vi "tfyghj.vi"() -> ()   [LabVIEW 2021]
uses:
  <vilib>/Platform/TimedLoop/XDataNode/timing_clust.ctl
  <vilib>/Platform/TimedLoop/XDataNode/nitl_modes.ctl
  <vilib>/Platform/TimedLoop/XDataNode/wakeup.ctl
  <vilib>/rvi/Emulation/niFpgaGetClockAttributes.vi
  <vilib>/rvi/Emulation/niFpgaSctlEmulationGetInTimedLoop.vi
  <vilib>/rvi/Emulation/niFpgaEmulationReportErrorSimple.vi
  <vilib>/rvi/Emulation/niFpgaCriticalErrorInLSC.vi
  <vilib>/platform/TimedLoop/XDataNode/XDataNode.xnode
  <vilib>/Platform/TimedLoop/XDataNode/XDNodeRunTimeDep.lvlib
panel:
  out "lut value at index":i16
  in  "Math":bool
  in  "PUT DIFFERENCE":i32
  out "Saw tooth \nactual freq":fxp<+,32,16>
  out "needed pre conversion":fxp<+,32,16>
  in  "Frequency":i32
  out "ticks needed post conversion":fxp<+/-,64,34>
  in  "SET DESIRED TICK":u32
  in  "Sin":bool
  out "sine out 3":i16
  out "sine out 2":i16
  out "sine out":i16
  out "C":bool
  out "B":bool
  out "Index":i32
  out "Difference Between":u32
  out "Current Time":u32
  out "Previous Time":u32
  out "A":bool
  out "Tick Count(Ticks)":u32
  in  "main":bool
  # "HOW TO USE:\n1) set desired SIN frequency\n2) the outputted ticks needed will be provided \nto find a frequency for the sawtooth ath is minimum 15x greater!\n!!!\nIF YOU PUT A DESIRED TICK SMALLER THAN THE NEEDED IT WILL\nPROVIDE A HIGHER FREQUENCY , A LARGER WILL BE SMALLER\n!!!"
  # "This is to calculate the actual frequency, put inside the difference\nto see what our lookup tabe output is actualy being worked at"
  # "IGNORE FOR NOW!!! HAVENT IMPLEMENTED\nchecks comparison of carrier and sin"
  # "This just reads out \nvalues from sin wave"
  # "Checks index and LUT values"
  # "WHere difference is derived"
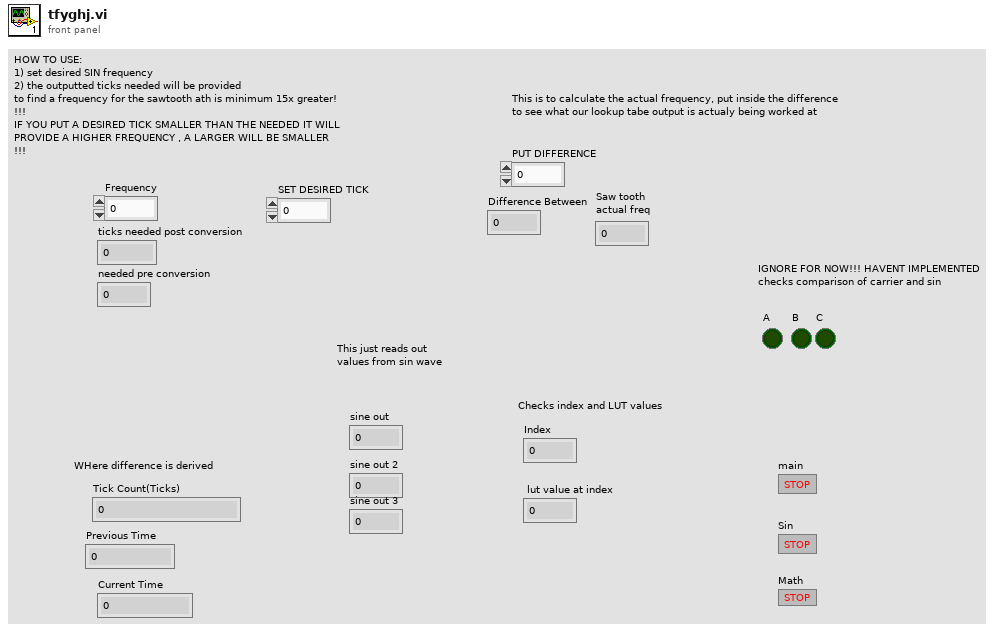
[diagram p1: front panel]
types:
  T1 = typedef "XDNodeRunTimeDep.lvlib/timing_clust.ctl" = cluster{"Expected End [f-1]":u64, "Actual End [f-1]":u64, "Finished Late? [f-1]":bool, "Expected End [i-1]":u64, "Actual End [i-1]":u64, "Finished Late? [i-1]":bool, "Expected Start [i]":u64, "Actual Start [i]":u64, "Expected Start [f]":u64, "Actual Start [f]":u64, "Source Name":string, "Structure Name":string, "Period":i64, "Deadline":i64, "Offset":i64, "Start":i64, "Priority":i32, "Timeout":i32, "Mode":T2, "Wakeup Reason":T3, "Error":errorcluster, "Source Type":string, "Secondary Source Type":string, "Global End Time":u64, "Global Start Time":u64, "Frame Duration":u64, "Iteration Duration":u64, "Assigned CPU":i32, "I/O Scan Engine Mode":u32}
  T2 = typedef "XDNodeRunTimeDep.lvlib/nitl_modes.ctl" = enum32{"No Change", "Process missed periods, maintain original phase", "Discard missed periods, maintain original phase", "Process missed periods, ignore original phase", "Discard missed periods, ignore original phase"}
  T3 = typedef "XDNodeRunTimeDep.lvlib/wakeup.ctl" = enum32{"Normal", "Aborted", "Asynchronous wakeup", "Timing source error", "Timed loop error", "Timeout"}
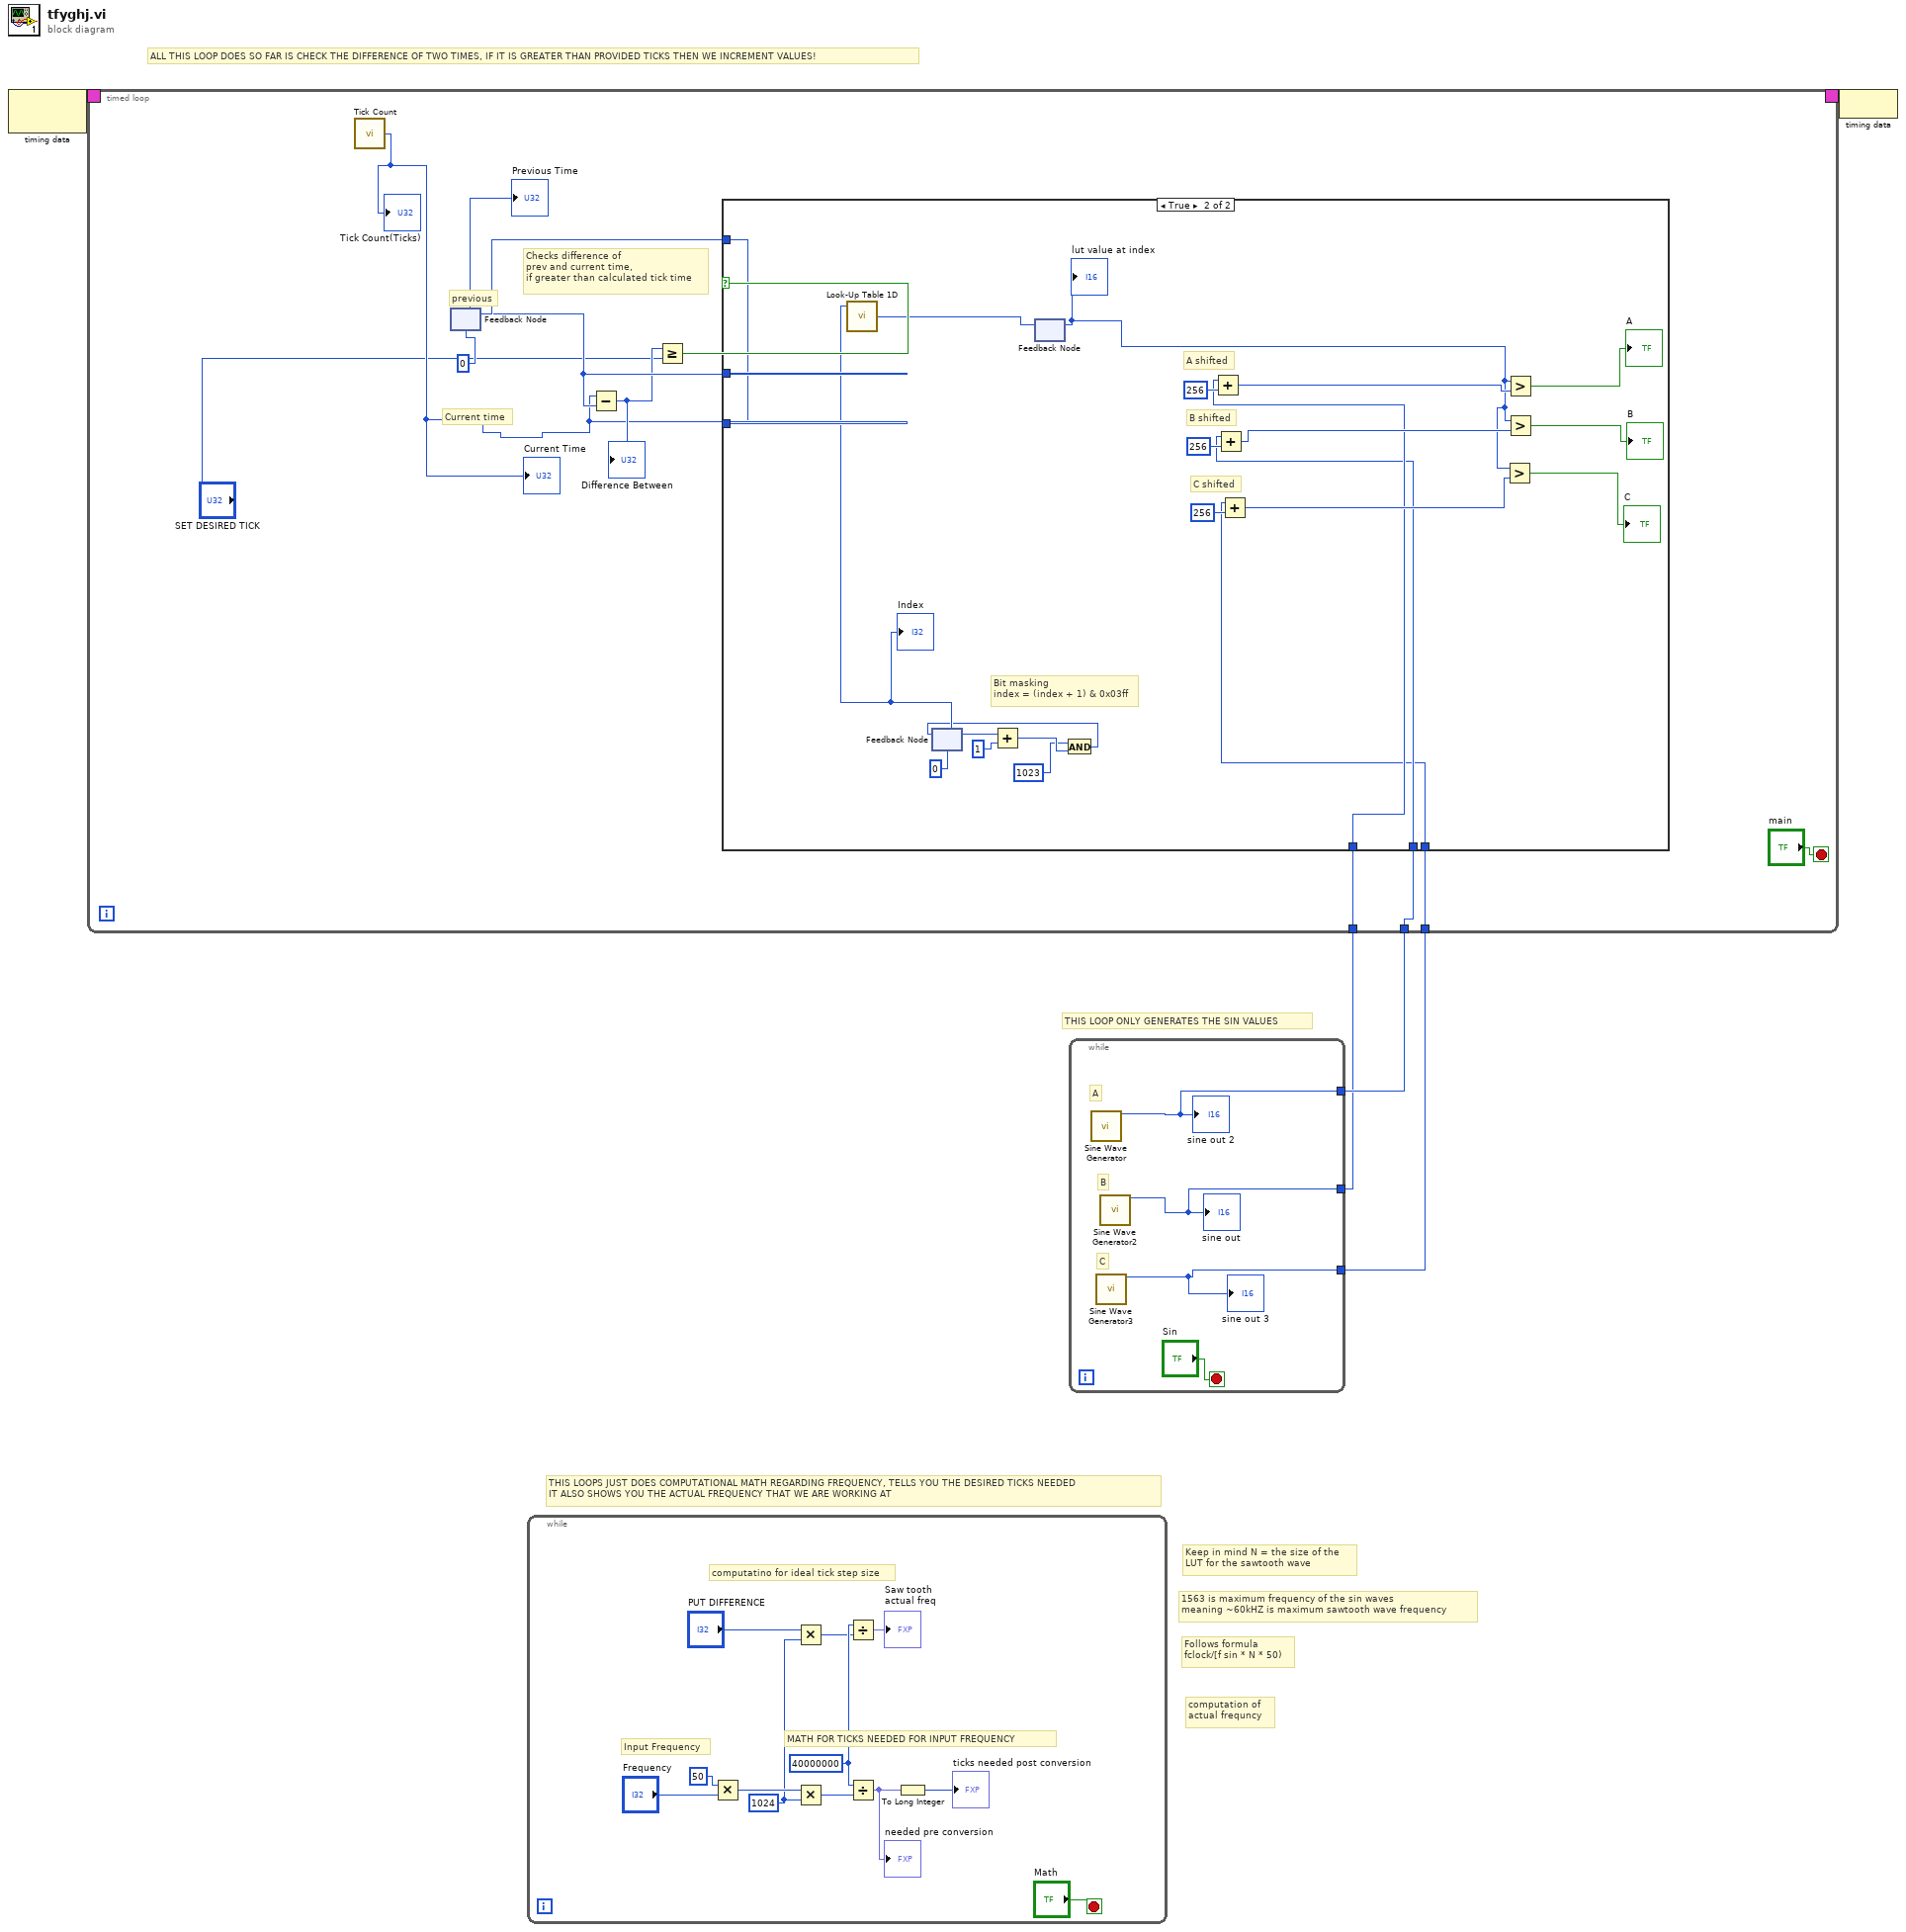
[diagram p0: block diagram]
diagram:
  # "ALL THIS LOOP DOES SO FAR IS CHECK THE DIFFERENCE OF TWO TIMES, IF IT IS GREATER THAN PROVIDED TICKS THEN WE INCREMENT VALUES!"
  # "computation of \nactual frequncy"
  # "1563 is maximum frequency of the sin waves \nmeaning ~60kHZ is maximum sawtooth wave frequency"
  # "Keep in mind N = the size of the \nLUT for the sawtooth wave"
  # "Follows formula \nfclock/[f sin * N * 50)"
  # "THIS LOOPS JUST DOES COMPUTATIONAL MATH REGARDING FREQUENCY, TELLS YOU THE DESIRED TICKS NEEDED\nIT ALSO SHOWS YOU THE ACTUAL FREQUENCY THAT WE ARE WORKING AT"
  # "THIS LOOP ONLY GENERATES THE SIN VALUES"
  n1 = node-c288() -> (w5:T1)  [unwired: 1 in]
  n2 = while {
    stop <- "Math" stop-if-true
    w11 = 1024
    w12 = 40000000
    # "MATH FOR TICKS NEEDED FOR INPUT FREQUENCY"
    # "computatino for ideal tick step size"
    # "Input Frequency"
    n3 = Multiply(x=50, y="Frequency") -> (x*y=w16:i32)
    n4 = Multiply(x="PUT DIFFERENCE", y=w11) -> (x*y=w10:u32)
    n5 = Multiply(x=w16, y=w11) -> (x*y=w15:i32)
    n6 = Divide(x=w12, y=w10) -> (x/y=→"Saw tooth \nactual freq":fxp<+,32,16>)
    n7 = Divide(x=w12, y=w15) -> (x/y=w14:fxp<+,32,16>)
    "needed pre conversion" <- w14
    n8 = To Long Integer(number=w14) -> (32bit integer=→"ticks needed post conversion":i32)
  }
  n9 = while {
    tunnel: [w20] -> w3
    tunnel: [w19] -> w2
    tunnel: [w18] -> w1
    stop <- "Sin" stop-if-true
    # "C"
    # "A"
    # "B"
    n10 = call "Sine Wave Generator"() -> ("sine out"=w20:i16)  [unwired: 15 in]
    "sine out 2" <- w20
    n11 = call "Sine Wave Generator3"() -> ("sine out"=w18:i16)  [unwired: 15 in]
    "sine out 3" <- w18
    n12 = call "Sine Wave Generator2"() -> ("sine out"=w19:i16)  [unwired: 15 in]
    "sine out" <- w19
  }
  n13 = timed-loop {
    timing: w5 -> [_]
    timing-out: [_] -> w4
    tunnel: w3 -> [w23]
    tunnel: w2 -> [w24]
    tunnel: w1 -> [w22]
    stop <- "main" stop-if-true
    # "Checks difference of \nprev and current time, \nif greater than calculated tick time"
    # "previous"
    # "Current time"
    n14 = call "Tick Count"() -> ("Tick Count(Ticks)"=w26:u32)
    "Tick Count(Ticks)" <- w26
    "Current Time" <- w26
    n15 = feedback #1(u32 0 ("Tick Count(Ticks)")) -> (w29:u32)
    "Previous Time" <- w29
    n16 = Subtract(x=w26, y=w29) -> (x-y=w27:u32)
    "Difference Between" <- w27
    n17 = Greater Or Equal?(x=w27, y="SET DESIRED TICK") -> (x >= y?=w31:bool)
    n18 = case shown="True" w31 {
      tunnel: w26 -> [_ w53]
      tunnel: [w33 w53] -> w30
      tunnel: w29 -> [w33 _]
      tunnel: w24 -> [_ w36]
      tunnel: w23 -> [_ w35]
      tunnel: w22 -> [_ w34]
      frame False {
      }
      frame True {
        # "Bit masking \nindex = (index + 1) & 0x03ff"
        # "C shifted"
        # "B shifted"
        # "A shifted"
        n19 = feedback #2(i16 0) -> (w40:i16)
        "Index" <- w40
        n20 = call "Look-Up Table 1D"("address"=w40) -> ("data out"=w43:i16)  [unwired: 8 in]
        n21 = Add(x=w40, y=i16 1) -> (x+y=w39:i16)
        n22 = feedback #3() -> (w42:i16)  [unwired: 1 in]
        "lut value at index" <- w42
        n23 = feedback-in #3(w43) -> ()
        n24 = And(x=i16 1023, y=w39) -> (x .and. y?=w37:i16)
        n25 = feedback-in #2(w37) -> ()
        n26 = Add(x=w36, y=u32 256) -> (x+y=w47:u32)
        n27 = Add(x=w35, y=u32 256) -> (x+y=w48:u32)
        n28 = Add(x=w34, y=u64 256) -> (x+y=w49:u64)
        n29 = Greater?(x=w42, y=w49) -> (0:→"C":bool)
        n30 = Greater?(x=w42, y=w47) -> (0:→"A":bool)
        n31 = Greater?(x=w42, y=w48) -> (0:→"B":bool)
      }
    }
    n32 = feedback-in #1(w30) -> ()
  }
  n33 = node-c288(w4) -> ()
